vi "Main.vi"() -> ()   [LabVIEW 2020]
doc: "This template is for the Queued Message Handler design pattern.\n\nThe Event Handling Loop generates messages based on user interface actions.\n\nThe Message Handling Loop processes messages generated by the Event Handling Loop, or by other messages. The messages are string values, so new messages can be added easily to the Message Cases case structure in the Message Handling Loop. Each message cluster can also provide an optional value for Message Data, which is a variant that can be converted to whatever message-specific data is required."
uses:
  <vilib>/vision/Image Controls.llb/IMAQ Image.ctl
  support/Message Queue/Enqueue Message (Single).vi
  <vilib>/Utility/error.llb/Error Cluster From Error Code.vi
  <vilib>/ErrorRing/Error Ring.xnode
  support/Message Queue/Message Queue.lvlib
  support/User Event - Stop/User Event - Stop.lvlib
panel:
  in  "Configurações":T1={"Simulações"={"Nível Qualidade"="avi", "Turno"="avi"}, "Captura de Imagens"={"Pasta com imagens"=path "", "Mostrar imagens capturadas"=FALSE}, "Caminhos"={"Arquivo de log"=path ""}}
  out "Qualidade atual":string="Ótima"
  out "Turno":string="Turno 1"
  out "Time Stamp":timestamp format="%<%X %x>T"
  out "Display":string
  in  "Sair":bool
  in  "Tab Control":T2(tab)
  in  "Iniciar Captura":bool
  out "Image Out":T3(plugin-control)
  in  "Configurações Avançadas":bool
  # "QUALIDADE:"
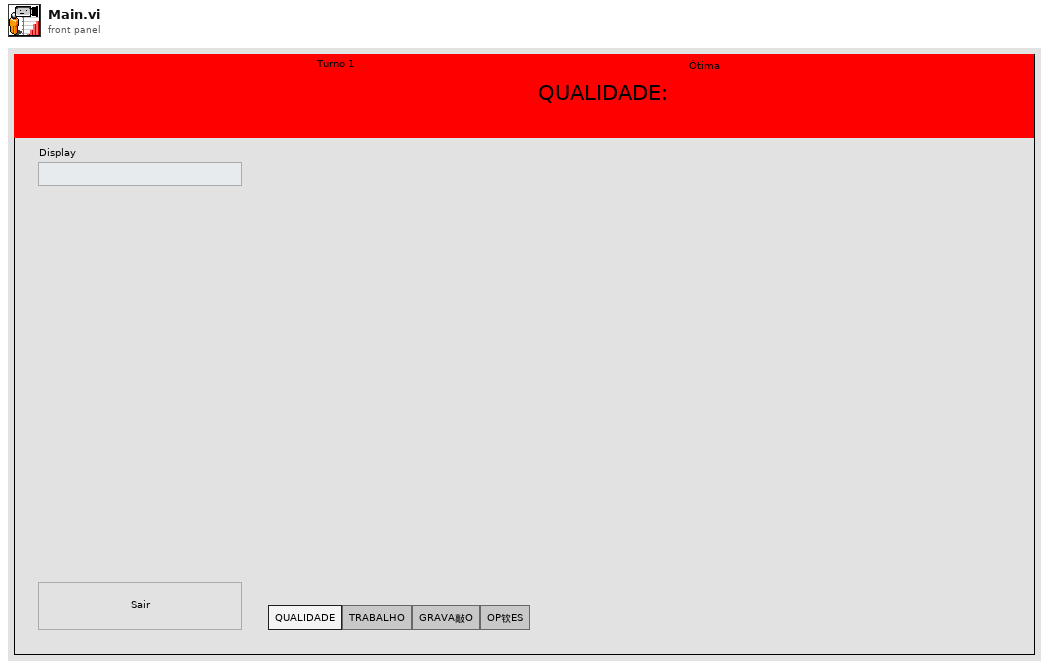
[diagram p1: front panel]
types:
  T1 = typedef "Configurações.lvlib/Configurações padrões.ctl" = cluster{"Simulações":cluster{"Nível Qualidade":string, "Turno":string}, "Captura de Imagens":cluster{"Pasta com imagens":path, "Mostrar imagens capturadas":bool}, "Caminhos":cluster{"Arquivo de log":path}}
  T2 = enum32{"QUALIDADE", "TRABALHO", "GRAVA敲O", "OP钦ES"}
  T3 = typedef "IMAQ Image.ctl" = refnum<image>
  T4 = enum16{"open", "replace", "create", "open or create", "replace or create", "replace or create with confirmation"}
  T5 = typedef "Message Queue.lvlib/All Message Queues.ctl" = cluster{"UI":refnum<queue>}
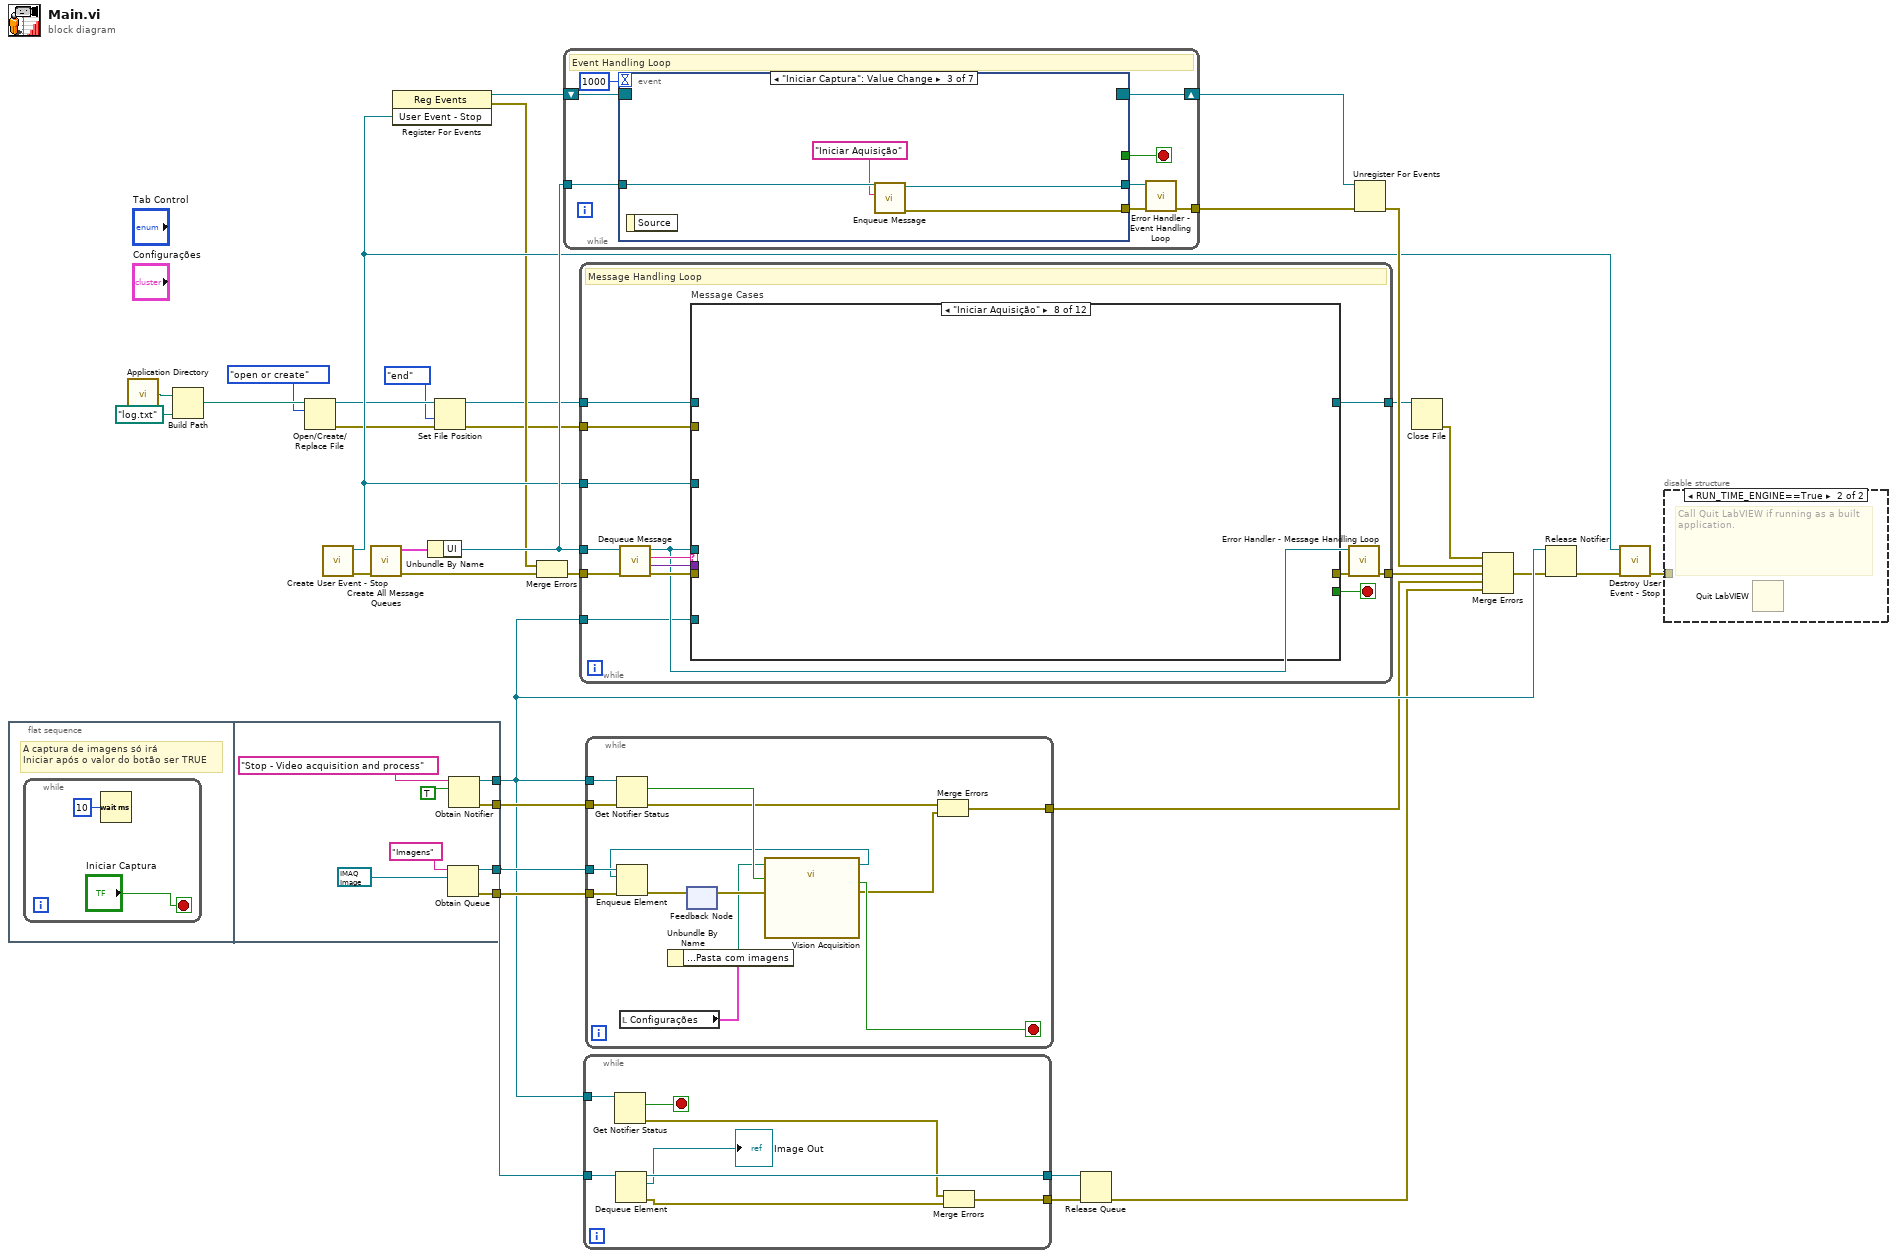
[diagram p0: block diagram]
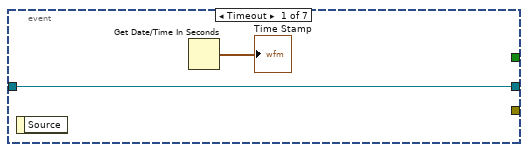
[diagram p3: hidden frame]
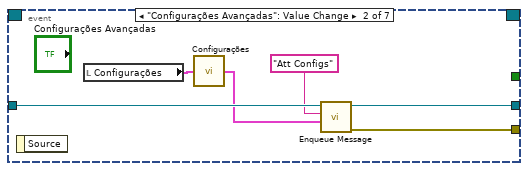
[diagram p4: hidden frame]
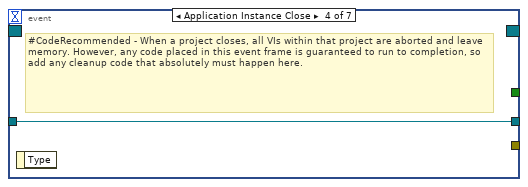
[diagram p5: hidden frame]
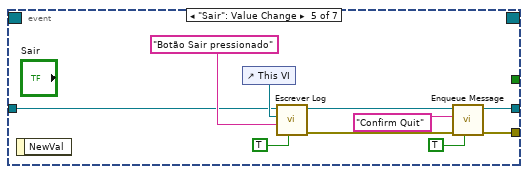
[diagram p6: hidden frame]
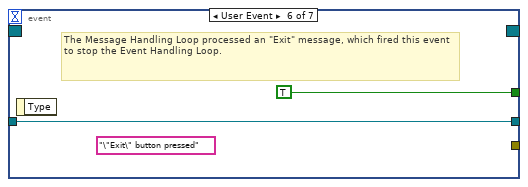
[diagram p7: hidden frame]
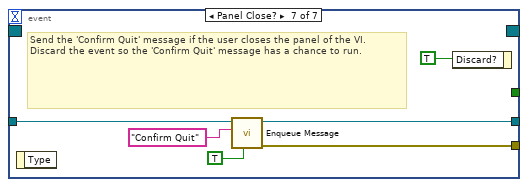
[diagram p8: hidden frame]
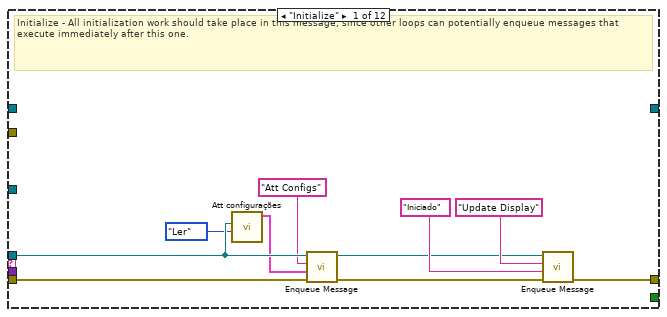
[diagram p9: hidden frame]
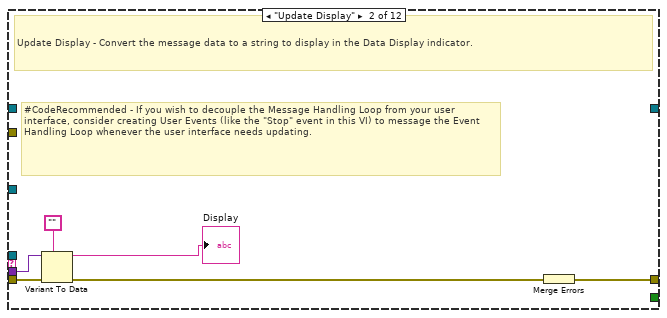
[diagram p10: hidden frame]
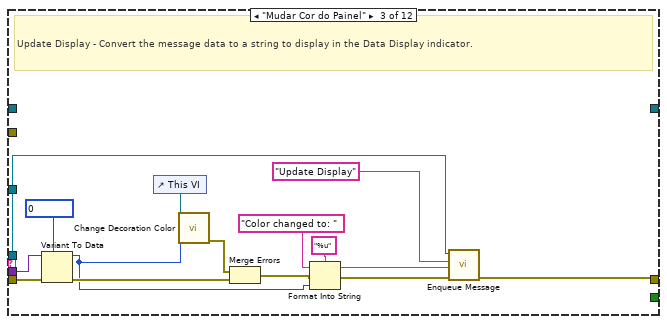
[diagram p11: hidden frame]
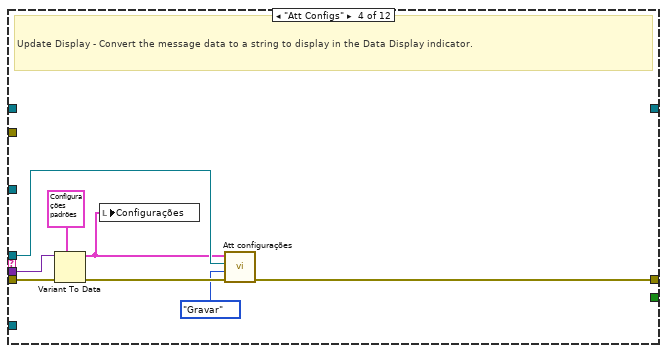
[diagram p12: hidden frame]
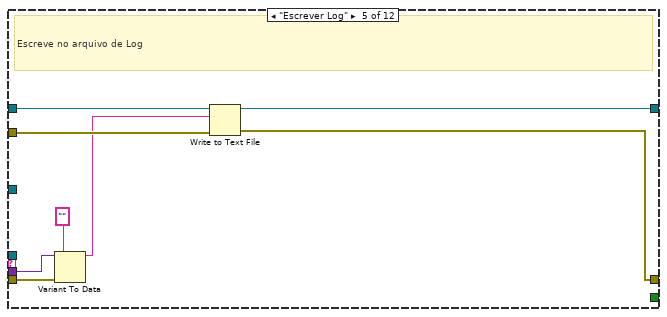
[diagram p13: hidden frame]
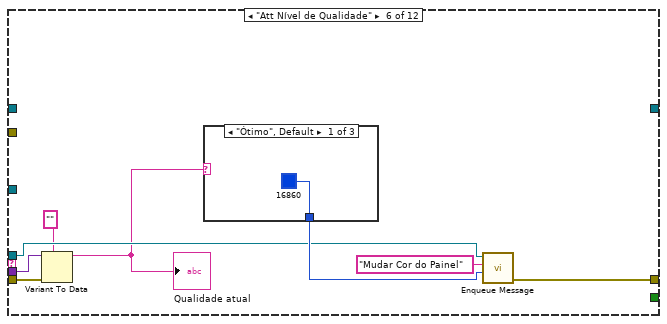
[diagram p14: hidden frame]
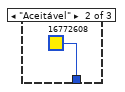
[diagram p15: hidden frame]
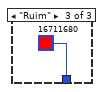
[diagram p16: hidden frame]
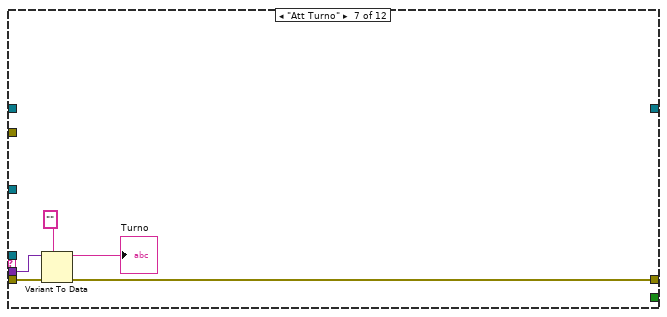
[diagram p17: hidden frame]
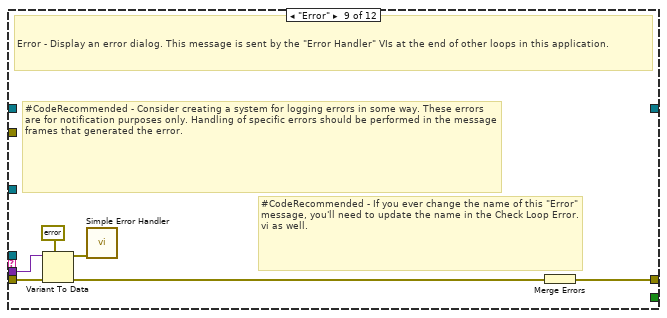
[diagram p18: hidden frame]
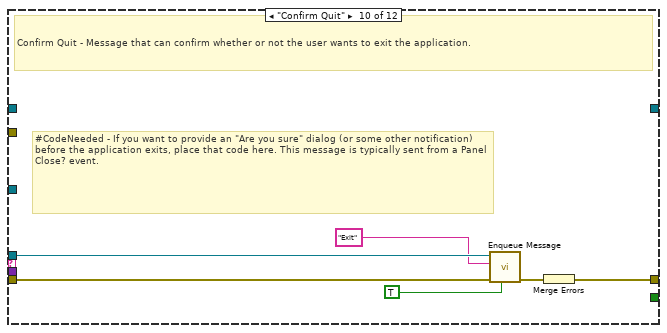
[diagram p19: hidden frame]
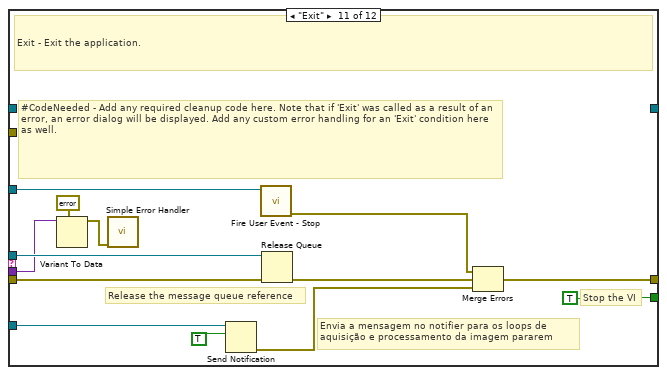
[diagram p20: hidden frame]
diagram:
  n1 = flat-sequence {
    tunnel: [w42] -> w21
    tunnel: [w41] -> w20
    tunnel: [w40] -> w19
    tunnel: [w39] -> w16
    frame #0 {
      # "A captura de imagens só irá\nIniciar após o valor do botão ser TRUE"
      n2 = while {
        stop <- "Iniciar Captura" stop-if-true
        n3 = Wait (ms)(milliseconds to wait=u32 10) -> ()  [unwired: 1 out]
      }
    }
    frame #1 {
      n4 = Obtain Queue(name (unnamed)="Imagens", element data type=T3 refnum ("Image Out 2")) -> (queue out=w40:refnum<queue>, error out=w42:errorcluster)  [unwired: 3 in, 1 out]
      n5 = Obtain Notifier(name (unnamed)="Stop - Video acquisition and process", notification data type=TRUE) -> (notifier out=w39:refnum<notifier>, error out=w41:errorcluster)  [unwired: 2 in, 1 out]
    }
  }
  n6 = call <vilib>:"Application Directory.vi"() -> ("Application Directory"=w9:path)
  n7 = Build Path(base path=w9, name or relative path=path "log.txt") -> (appended path=w8:path)
  n8 = Open/Create/Replace File(file path (use dialog)=w8, operation (0:open)=T4."open or create") -> (refnum out=w5:refnum<file>, error out=w3:errorcluster)  [unwired: 4 in, 1 out]
  n9 = call "Create User Event - Stop.vi"() -> ("error out"=w30:errorcluster, "User Event - Stop"=w24:refnum<user-event>)  [unwired: 10 in]
  n10 = call "Create All Message Queues.vi"("error in (no error)"=w30) -> ("error out"=w34:errorcluster, "Message Queues out"=w33:T5)  [unwired: 9 in]
  n11 = register-events(w24) -> (reference out=w25:refnum<event-registration>, error out=w22:errorcluster)  [unwired: 2 in]
  n12 = Unbundle By Name(w33) -> ("UI"=w31:refnum<queue>)
  n13 = Set File Position(refnum=w5, from (0:start)=enum16{"start", "end", "current"}."end", error in=w3) -> (refnum out=w4:refnum<file>, error out=w2:errorcluster)  [unwired: 1 in]
  n14 = Merge Errors(w22, w34) -> (w23:errorcluster)
  n15 = while {
    tunnel: w31 -> [w52]
    shift-right: [w50] -> w28
    shift-left: w25 -> [w51]
    tunnel: [w46] -> w26
    stop <- w48 stop-if-true
    # "Event Handling Loop"
    n16 = event shown="[2] \"Iniciar Captura\": Value Change" {
      selector: w51 -> [_ _ _ _ _ _ _]
      dyn-events: [_ _ _ _ _ _ _] -> w50
      timeout: 1000 -> [_ _ _ _ _ _ _]
      tunnel: [_ _ _ _ _ TRUE ("Discard?") _] -> w48
      tunnel: w52 -> [w54 w59 w64 w65 w70 w77 w82]
      tunnel: [_ w58 w62 _ w66 _ w81] -> w49
      tunnel: [w54 w60 w63 w65 w68 w77 w80] -> w47
      event Timeout {
        n17 = event-data() -> ()  [unwired: 1 in, 1 out]
        n18 = Get Date/Time In Seconds() -> (seconds since 1Jan1904=→"Time Stamp":timestamp)
      }
      event "Configurações Avançadas": Value Change {
        n19 = event-data() -> ()  [unwired: 1 in, 1 out]
        n20 = local read "Configurações"() -> (w55:T1)
        n21 = call "Configurações.vi"("Configurações"=w55) -> ("Saída de Configurações"=w57:T1)
        n22 = call-poly "Enqueue Message.vi"("Message Data"=w57, "Message"="Att Configs", "Message Queue"=w59) -> ("error out"=w58:errorcluster, "dup Message Queue"=w60:refnum<queue>)  [unwired: 7 in]
      }
      event "Iniciar Captura": Value Change {
        n23 = event-data() -> ()  [unwired: 1 in, 1 out]
        n24 = call-poly "Enqueue Message.vi"("Message"="Iniciar Aquisição", "Message Queue"=w64) -> ("error out"=w62:errorcluster, "dup Message Queue"=w63:refnum<queue>)  [unwired: 8 in]
      }
      event Application Instance Close {
        # "#CodeRecommended - When a project closes, all VIs within that project are aborted and leave memory. However, any code placed in this event frame is guaranteed to run to completion, so add any cleanup code that absolutely must happen here."
        n25 = event-data() -> ()  [unwired: 1 in, 1 out]
      }
      event "Sair": Value Change {
        n26 = event-data() -> ()  [unwired: 1 in, 1 out]
        n27 = control-ref of="This VI"() -> (w73:refnum<vi>)
        n28 = call "Escrever Log.vi"("Priorizar mensagem"=TRUE, "Dados para Log"="Botão Sair pressionado", "VI"=w73, "Queue in"=w70) -> ("error out"=w67:errorcluster, "dup Message Queue"=w69:refnum<queue>)  [unwired: 6 in]
        n29 = call-poly "Enqueue Message.vi"("Priority Message? (F)"=TRUE, "error in (no error)"=w67, "Message"="Confirm Quit", "Message Queue"=w69) -> ("error out"=w66:errorcluster, "dup Message Queue"=w68:refnum<queue>)  [unwired: 6 in]
      }
      event User Event {
        (unwired) "\"Exit\" button pressed" ("VI Stopped")
        # "The Message Handling Loop processed an \"Exit\" message, which fired this event to stop the Event Handling Loop."
        n30 = event-data() -> ()  [unwired: 1 in, 1 out]
      }
      event Panel Close? {
        # "Send the 'Confirm Quit' message if the user closes the panel of the VI. Discard the event so the 'Confirm Quit' message has a chance to run."
        n31 = event-data() -> ()  [unwired: 1 in, 1 out]
        n32 = call-poly "Enqueue Message.vi"("Priority Message? (F)"=TRUE, "Message"="Confirm Quit", "Message Queue"=w82) -> ("error out"=w81:errorcluster, "dup Message Queue"=w80:refnum<queue>)  [unwired: 7 in]
        n33 = event-data("Discard?"=TRUE) -> ()  [unwired: 1 in, 1 out]
      }
    }
    n34 = call "Error Handler - Event Handling Loop.vi"("error in (no error)"=w49, "Message Queue"=w47) -> ("dup error in"=w46:errorcluster)  [unwired: 8 in, 1 out]
  }
  n35 = while {
    tunnel: w31 -> [w91]
    tunnel: w24 -> [w96]
    tunnel: w23 -> [w95]
    tunnel: [w89] -> w32
    tunnel: w16 -> [w87]
    tunnel: w4 -> [w86]
    tunnel: [w85] -> w11
    tunnel: w2 -> [w84]
    stop <- w97 stop-if-true
    # "Message Handling Loop"
    n36 = call "Dequeue Message.vi"("error in (no error)"=w95, "Message Queue"=w91) -> ("error out"=w94:errorcluster, "Message Data"=w92:variant, "Message"=w93:string, "dup Message Queue"=w90:refnum<queue>)  [unwired: 6 in]
    n37 = case "Message Cases" shown="\"Iniciar Aquisição\"" w93 {
      selector: w93 -> [_ _ _ _ _ _ _ _ _ _ _ w186]
      tunnel: w90 -> [w101 _ w122 w131 _ w147 _ _ _ w169 w185 _]
      tunnel: w94 -> [w103 w112 w128 w136 w144 w152 w160 _ w166 w172 w179 _]
      tunnel: [w107 w113 w123 w132 w137 w150 w156 _ w161 w171 w182 w187] -> w88
      tunnel: [_ _ _ _ _ _ _ _ _ _ TRUE _] -> w97
      tunnel: w92 -> [_ w111 w127 w135 w143 w151 w159 _ w165 _ w176 _]
      tunnel: w96 -> [_ _ _ _ _ _ _ _ _ _ w181 _]
      tunnel: w87 -> [_ _ _ _ _ _ _ _ _ _ w175 _]
      tunnel: w86 -> [_ _ _ _ w141 _ _ _ _ _ _ _]
      tunnel: [_ _ _ _ w140 _ _ _ _ _ _ _] -> w85
      tunnel: w84 -> [_ _ _ _ w139 _ _ _ _ _ _ _]
      frame "Initialize" {
        # "Initialize - All initialization work should take place in this message, since other loops can potentially enqueue messages that execute immediately after this one."
        n38 = call "Att configurações.vi"("Message Queue"=w101, "Ler/Gravar"=enum16{"Ler", "Gravar"}."Ler") -> ("Saída de configurações"=w100:T1)  [unwired: 7 in, 1 out]
        n39 = call-poly "Enqueue Message.vi"("error in (no error)"=w103, "Message Data"=w100, "Message"="Att Configs", "Message Queue"=w101) -> ("error out"=w102:errorcluster, "dup Message Queue"=w104:refnum<queue>)  [unwired: 6 in]
        n40 = call-poly "Enqueue Message.vi"("error in (no error)"=w102, "Message Data"="Iniciado" ("Initial Message"), "Message"="Update Display", "Message Queue"=w104) -> ("error out"=w107:errorcluster)  [unwired: 6 in, 1 out]
      }
      frame "Update Display" {
        # "#CodeRecommended - If you wish to decouple the Message Handling Loop from your user interface, consider creating User Events (like the \"Stop\" event in this VI) to message the Event Handling Loop whenever the user interface needs updating."
        # "Update Display - Convert the message data to a string to display in the Data Display indicator."
        n41 = Variant To Data(error in=w112, type="", Variant=w111) -> (data=→"Display":string, error out=w109:errorcluster)
        n42 = Merge Errors(w109) -> (w113:errorcluster)
      }
      frame "Mudar Cor do Painel" {
        # "Update Display - Convert the message data to a string to display in the Data Display indicator."
        n43 = Variant To Data(error in=w128, type=u32 0 ("Colors:BG Color"), Variant=w127) -> (data=w115:u32, error out=w126:errorcluster)
        n44 = control-ref of="This VI"() -> (w114:refnum<vi>)
        n45 = call "Change Decoration Color.vi"("This VI"=w114, "Colors:BG Color"=w115) -> ("error out"=w124:errorcluster)  [unwired: 8 in]
        n46 = Merge Errors(w124, w126) -> (w120:errorcluster)
        n47 = Format Into String(format string="%u", initial string="Color changed to: ", error in=w120, w115) -> (resulting string=w117:string, error out=w119:errorcluster)
        n48 = call-poly "Enqueue Message.vi"("error in (no error)"=w119, "Message Data"=w117, "Message"="Update Display", "Message Queue"=w122) -> ("error out"=w123:errorcluster)  [unwired: 6 in, 1 out]
      }
      frame "Att Configs" {
        # "Update Display - Convert the message data to a string to display in the Data Display indicator."
        n49 = Variant To Data(error in=w136, type=T1 {"Simulações"={"Nível Qualidade"="Ótima", "Turno"="Turno 1"}, "Captura de Imagens"={"Pasta com imagens"=path "", "Mostrar imagens capturadas"=FALSE}, "Caminhos"={"Arquivo de log"=path ""}} ("Configurações"), Variant=w135) -> (data=w129:T1, error out=w133:errorcluster)
        n50 = local write "Configurações"(w129) -> ()
        n51 = call "Att configurações.vi"("Entrada de Configurações"=w129, "Message Queue"=w131, "Ler/Gravar"=enum16{"Ler", "Gravar"}."Gravar", "error in (no error)"=w133) -> ("error out"=w132:errorcluster)  [unwired: 5 in, 1 out]
      }
      frame "Escrever Log" {
        # "Escreve no arquivo de Log"
        n52 = Variant To Data(error in=w144, type="" ("string"), Variant=w143) -> (data=w138:string)  [unwired: 1 out]
        n53 = Write to Text File(file (use dialog)=w141, text=w138, error in=w139) -> (refnum out=w140:refnum<file>, error out=w137:errorcluster)  [unwired: 1 in, 1 out]
      }
      frame "Att Nível de Qualidade" {
        n54 = Variant To Data(error in=w152, type="", Variant=w151) -> (data=w145:string)  [unwired: 1 out]
        "Qualidade atual" <- w145
        n55 = case shown="\"Ótimo\", Default" w145 {
          tunnel: [u32 16860 u32 16772608 u32 16711680] -> w148
          frame "Ótimo", Default {
          }
          frame "Aceitável" {
          }
          frame "Ruim" {
          }
        }
        n56 = call-poly "Enqueue Message.vi"("Message Data"=w148, "Message"="Mudar Cor do Painel", "Message Queue"=w147) -> ("error out"=w150:errorcluster)  [unwired: 7 in, 1 out]
      }
      frame "Att Turno" {
        n57 = Variant To Data(error in=w160, type="", Variant=w159) -> (data=→"Turno":string, error out=w156:errorcluster)
      }
      frame "Iniciar Aquisição" {
      }
      frame "Error" {
        # "#CodeRecommended - If you ever change the name of this \"Error\" message, you'll need to update the name in the Check Loop Error.vi as well."
        # "#CodeRecommended - Consider creating a system for logging errors in some way. These errors are for notification purposes only. Handling of specific errors should be performed in the message frames that generated the error."
        # "Error - Display an error dialog. This message is sent by the \"Error Handler\" VIs at the end of other loops in this application."
        n58 = Variant To Data(error in=w166, type=errorcluster {"status"=FALSE, "code"=0, "source"=""} ("error constant"), Variant=w165) -> (data=w163:errorcluster, error out=w162:errorcluster)
        n59 = call <vilib>:"Simple Error Handler.vi"("error in (no error)"=w163) -> ()  [unwired: 4 in, 5 out]
        n60 = Merge Errors(w162) -> (w161:errorcluster)
      }
      frame "Confirm Quit" {
        # "#CodeNeeded - If you want to provide an \"Are you sure\" dialog (or some other notification) before the application exits, place that code here. This message is typically sent from a Panel Close? event."
        # "Confirm Quit - Message that can confirm whether or not the user wants to exit the application."
        n61 = call-poly "Enqueue Message.vi"("Priority Message? (F)"=TRUE, "error in (no error)"=w172, "Message"="Exit", "Message Queue"=w169) -> ("error out"=w170:errorcluster)  [unwired: 6 in, 1 out]
        n62 = Merge Errors(w170) -> (w171:errorcluster)
      }
      frame "Exit" {
        # "Envia a mensagem no notifier para os loops de\naquisição e processamento da imagem pararem"
        # "Stop the VI"
        # "Release the message queue reference"
        # "#CodeNeeded - Add any required cleanup code here. Note that if 'Exit' was called as a result of an error, an error dialog will be displayed. Add any custom error handling for an 'Exit' condition here as well."
        # "Exit - Exit the application."
        n63 = Variant To Data(type=errorcluster {"status"=FALSE, "code"=0, "source"=""} ("error constant"), Variant=w176) -> (data=w177:errorcluster)  [unwired: 1 in, 1 out]
        n64 = call <vilib>:"Simple Error Handler.vi"("error in (no error)"=w177) -> ()  [unwired: 4 in, 5 out]
        n65 = Send Notification(notification=TRUE, notifier=w175) -> (error out=w173:errorcluster)  [unwired: 1 in, 1 out]
        n66 = call "Fire User Event - Stop.vi"("User Event - Stop"=w181) -> ("error out"=w180:errorcluster)  [unwired: 10 in]
        n67 = Release Queue(queue=w185, error in (no error)=w179) -> (error out=w183:errorcluster)  [unwired: 1 in, 2 out]
        n68 = Merge Errors(w180, w183, w173) -> (w182:errorcluster)
      }
      frame Default {
        # "'Default' case only runs if there is a message that isn't defined in any of the other cases.  Output a programming error."
        n69 = xnode "Error Ring"("parameter 0"=w186) -> ("error out"=w187:errorcluster)
      }
    }
    n70 = call "Error Handler - Message Handling Loop.vi"("error in (no error)"=w88, "Message Queue"=w90) -> ("dup error in"=w89:errorcluster)  [unwired: 8 in, 1 out]
  }
  n71 = while {
    tunnel: w16 -> [w202]
    tunnel: w19 -> [w200]
    tunnel: [w199] -> w18
    tunnel: [w197] -> w17
    stop <- w201 stop-if-true
    n72 = Get Notifier Status(notifier=w202) -> (current notification=w201:bool, error out=w195:errorcluster)  [unwired: 1 in, 3 out]
    n73 = Dequeue Element(queue=w200) -> (queue out=w199:refnum<queue>, element=→"Image Out":T3, error out=w196:errorcluster)  [unwired: 2 in, 1 out]
    n74 = Merge Errors(w195, w196) -> (w197:errorcluster)
  }
  n75 = while {
    tunnel: w16 -> [w216]
    tunnel: w19 -> [w214]
    tunnel: w21 -> [w207]
    tunnel: w20 -> [w206]
    tunnel: [w205] -> w15
    stop <- w212 stop-if-true
    n76 = Get Notifier Status(notifier=w216, error in (no error)=w206) -> (current notification=w215:bool, error out=w209:errorcluster)  [unwired: 3 out]
    n77 = local read "Configurações"() -> (w204:T1)
    n78 = Unbundle By Name(w204) -> ("Captura de Imagens.Pasta com imagens"=w203:path)
    n79 = feedback #1() -> (w210:errorcluster)  [unwired: 1 in]
    n80 = call "Vision Acquisition"("Image Path"=w203, "Stop (F)"=w215, "error in"=w210) -> ("Image Out"=w213:T3, "Stopped"=w212:bool, "error out"=w208:errorcluster)  [unwired: 21 in, 1 out]
    n81 = Enqueue Element(queue=w214, element=w213, error in (no error)=w207) -> (error out=w211:errorcluster)  [unwired: 1 in, 2 out]
    n82 = feedback-in #1(w211) -> ()
    n83 = Merge Errors(w209, w208) -> (w205:errorcluster)
  }
  n84 = Release Queue(queue=w18, error in (no error)=w17) -> (error out=w14:errorcluster)  [unwired: 1 in, 2 out]
  n85 = Unregister For Events(event registration refnum=w28, error in=w26) -> (error out=w29:errorcluster)
  n86 = Close File(refnum=w11) -> (error out=w10:errorcluster)  [unwired: 1 in, 1 out]
  n87 = Merge Errors(w10, w29, w32, w15, w14) -> (w13:errorcluster)
  n88 = Release Notifier(notifier=w16, error in (no error)=w13) -> (error out=w12:errorcluster)  [unwired: 1 in, 2 out]
  n89 = call "Destroy User Event - Stop.vi"("error in (no error)"=w12, "User Event - Stop"=w24) -> ("error out"=w27:errorcluster)  [unwired: 9 in]
  n90 = disable-structure shown="RUN_TIME_ENGINE==True" {
    disable-tunnel: w27 -> [_ _]
    frame condition #0 (active) {
    }
    frame condition #1 {
      # "Call Quit LabVIEW if running as a built application."
      n91 = Quit LabVIEW() -> ()  [unwired: 1 in]
    }
  }
